vi "Spectrum.vi"(8 "error in (no error)":errorcluster) -> (0 "error out":errorcluster, 1 "Spectrum":dbl[](array[numeric]), 2 "Channel Scale":dbl[](array[numeric]), 3 "Channels":i32)   [LabVIEW 2018]
uses:
  SesWrapper/SesWrapper.lvlib
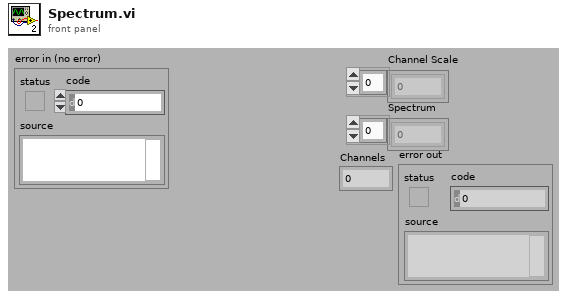
[diagram p1: front panel]
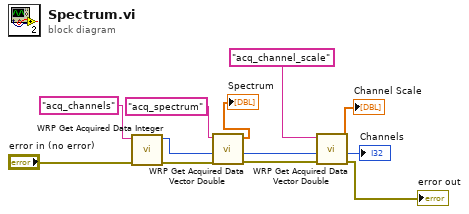
[diagram p0: block diagram]
diagram:
  n1 = call "WRP Get Acquired Data Integer.vi"("error in (no error)"="error in (no error)", "parameter"="acq_channels") -> ("error out"=w11:errorcluster, "data"=w2:i32)  [unwired: 6 in, 2 out]
  n2 = call "WRP Get Acquired Data Vector Double.vi"("error in (no error)"=w11, "size"=w2, "parameter"="acq_spectrum") -> ("error out"=w3:errorcluster, "size out"=w1:i32, "data"=→"Spectrum":dbl[])  [unwired: 5 in, 1 out]
  n3 = call "WRP Get Acquired Data Vector Double.vi"("error in (no error)"=w3, "size"=w1, "parameter"="acq_channel_scale") -> ("error out"=→"error out":errorcluster, "size out"=→"Channels":i32, "data"=→"Channel Scale":dbl[])  [unwired: 5 in, 1 out]
